vi "GetStreamingFilterIDs.vi"(8 "error in (no error)":errorcluster, 11 "Ref":T1) -> (0 "error out":errorcluster, 2 "IDs":u64[](array[numeric]), 3 "Ref":T1)   [LabVIEW 2019, in "Diagnostics Host Automation API.lvlib"]
uses:
  Diagnostics Host Automation API.lvlib
  Addon/Addon Shared/Types/HostAutomation.Ref.ctl
  <vilib>/NI/STM/TCP/TCP Connection Info.ctl
  <vilib>/NI/STM/SubVIs/MetaDataElement.ctl
  Addon/Addon Shared/Types/DTC.Codes.ctl
  <vilib>/NI/NI VeriStand Addon Network Comm/Shared/NI VeriStand Addon Network Comm Shared.lvlib
  <vilib>/NI/STM/NI STM.lvlib
  Addon/Addon Shared/Diagnostics Addon Shared.lvlib
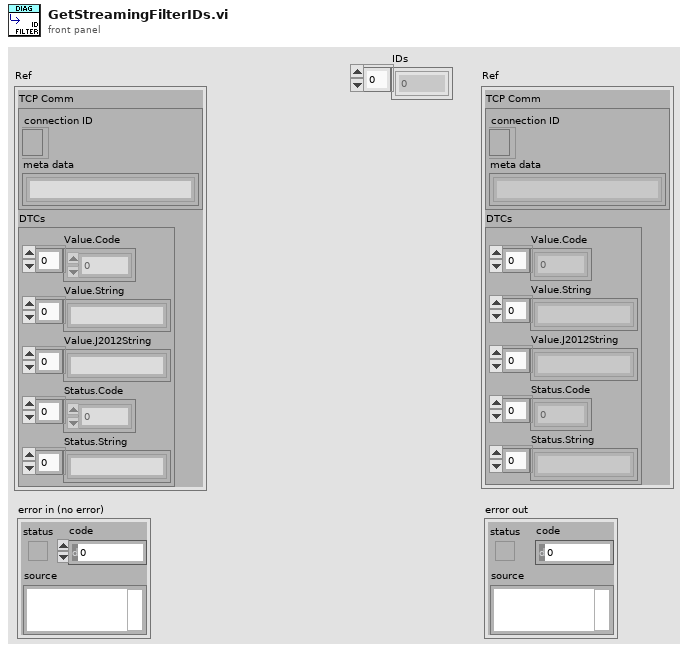
[diagram p1: front panel]
types:
  T1 = typedef "Diagnostics Addon Shared.lvlib/HostAutomation.Ref.ctl" = cluster{"TCP Comm":T2, "DTCs":T4}
  T2 = typedef "NI STM.lvlib/TCP Connection Info.ctl" = cluster{"connection ID":refnum<k5>, "meta data":T3[]}
  T3 = typedef "NI STM.lvlib/MetaDataElement.ctl" = string
  T4 = typedef "Diagnostics Addon Shared.lvlib/DTC.Codes.ctl" = cluster{"Value.Code":dbl[], "Value.String":string[], "Value.J2012String":string[], "Status.Code":dbl[], "Status.String":string[]}
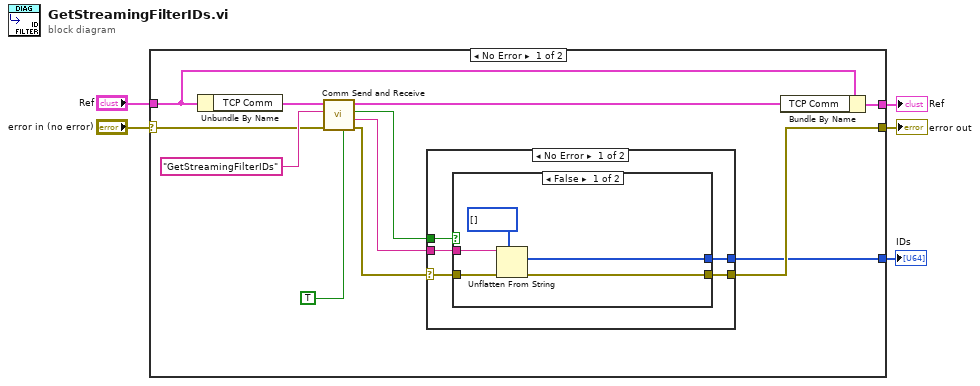
[diagram p0: block diagram]
diagram:
  n1 = case shown="No Error" "error in (no error)" {
    selector: "error in (no error)" -> [w7 w31]
    tunnel: "Ref" -> [w15 w30]
    tunnel: [w13 w30] -> w4
    tunnel: [w9 w31] -> w3
    tunnel: [w6 _] -> w1
    frame No Error {
      n2 = Unbundle By Name(w15) -> ("TCP Comm"=w16:T2)
      n3 = call <vilib>:"Comm Send and Receive.vi"("Resp Required?"=TRUE, "error in (no error)"=w7, "Name"="GetStreamingFilterIDs", "connection info"=w16) -> ("error out"=w10:errorcluster, "Data"=w12:string, "Timed Out?"=w11:bool, "connection info"=w14:T2)  [unwired: 4 in]
      n4 = case shown="No Error" w10 {
        selector: w10 -> [w20 w29]
        tunnel: w11 -> [w22 _]
        tunnel: [w21 w29] -> w9
        tunnel: w12 -> [w19 _]
        tunnel: [w18 _] -> w6
        frame No Error {
          n5 = case shown="False" w22 {
            tunnel: [w26 w28] -> w21
            tunnel: w20 -> [w27 w28]
            tunnel: w19 -> [w25 _]
            tunnel: [w23 _] -> w18
            frame False {
              n6 = Unflatten From String(type=u64[] [], binary string=w25, error in (no error)=w27) -> (value=w23:u64[], error out=w26:errorcluster)  [unwired: 2 in, 1 out]
            }
            frame True {
            }
          }
        }
        frame Error {
        }
      }
      n7 = Bundle By Name(cluster=w15, "TCP Comm"=w14) -> (w13:T1)
    }
    frame Error {
    }
  }
  "Ref" <- w4
  "error out" <- w3
  "IDs" <- w1
